vi "SendMessage.vi"(8 "error in (no error)":errorcluster, 10 "data in":string, 11 "STOMP in":refnum<class "STOMP.lvclass">) -> (0 "error out":errorcluster, 3 "STOMP out":refnum<class "STOMP.lvclass">)   [LabVIEW 2017, in "STOMP.lvclass"]
uses:
  STOMP.lvclass
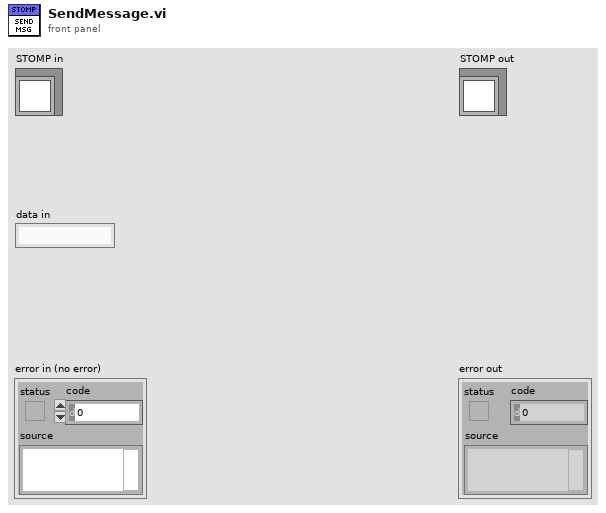
[diagram p1: front panel]
types:
  T1 = typedef "STOMP.lvclass/ObjectAttributes.ctl" = cluster{"address":string, "port":u16, "ConnectionRef":refnum<k5>, "messageQueue":refnum<queue>, "receiptQueue":refnum<queue>, "errorQueue":refnum<queue>, "sendQueue":refnum<queue>, "currentReceiptNumber":u64, "currentSubscriptionId":u64, "closeConnection":bool, "activeSubscriptions":T2[]}
  T2 = typedef "STOMP.lvclass/Type_ActiveSubscription.ctl" = cluster{"id":u64, "receipt":bool, "Destination":string, "ack":T3, "headers":T4[]}
  T3 = typedef "STOMP.lvclass/Type_AckHeader.ctl" = enum16{"auto", "client", "client-individual"}
  T4 = typedef "STOMP.lvclass/Type_FrameHeader.ctl" = cluster{"Header":string, "Value":string}
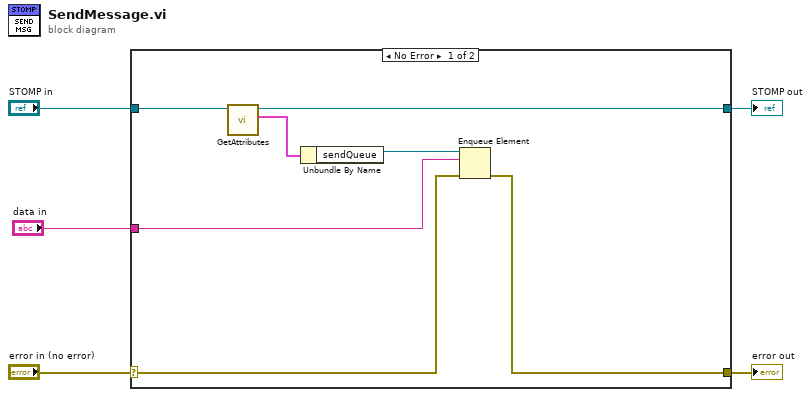
[diagram p0: block diagram]
diagram:
  n1 = case shown="No Error" "error in (no error)" {
    selector: "error in (no error)" -> [w10 w14]
    tunnel: [w9 w14] -> w4
    tunnel: [w6 w13] -> w2
    tunnel: "STOMP in" -> [w8 w13]
    tunnel: "data in" -> [w11 _]
    frame No Error {
      n2 = call-dynamic "GetAttributes.vi"("STOMP in"=w8) -> ("attributes"=w7:T1, "STOMP out"=w6:refnum<class "STOMP.lvclass">)  [unwired: 8 in, 1 out]
      n3 = Unbundle By Name(w7) -> ("sendQueue"=w12:refnum<queue>)
      n4 = Enqueue Element(queue=w12, element=w11, error in (no error)=w10) -> (error out=w9:errorcluster)  [unwired: 1 in, 2 out]
    }
    frame Error {
    }
  }
  "error out" <- w4
  "STOMP out" <- w2
